vi "Resize.Align Child Tab Ctrl within Parent Tab Ctrl.vi"(4 "Child Ref Pos":T1(ring), 5 "dY":i32, 6 "Parent Ref Pos":T1(ring), 7 "dX":i32, 8 "error in":errorcluster, 10 "Child Tab Ctrl":refnum<vi>, 11 "Parent Tab Ctrl":refnum<vi>) -> (0 "error out":errorcluster, 2 "Child Tab Ctrl Out":refnum<vi>, 3 "Parent Tab Ctrl Out":refnum<vi>)   [LabVIEW 2024, in "EQMF.lvlib" / "Controls.lvlib"]
doc: "This VI aligns a tab control (child) within another tab control (parent).\nThe inner control is moved to within Dx and Dy distance (in pixels) from the referenced corners specified by the inputs Parent Ref Pos and Child Ref Pos.\n\nINPUTS:\n<B>dX</B> - The delta X position.\n<B>dY</B> - The delta Y position.\n<B>Parent Tab Ctrl</B> - Control of the parent tab.\n<B>Child Tab Ctrl</B> - Control of the child tab.\n<B>Parent Ref Pos</B> - An enumerator specifying the corner that is to be aligned.\n<B>Child Ref Pos</B> - An enumerator specifying the corner that is to be aligned.\n\nOUTPUTS:\n<B>Parent Tab Ctrl</B> - Duplicate control of the parent tab.\n<B>Child Tab Ctrl</B> - Duplicate control of the child tab.\n\nERRORS: \nAn error will be generated if one of the controls are the incorrect type or if the control reference is invalid."
uses:
  Controls.lvlib
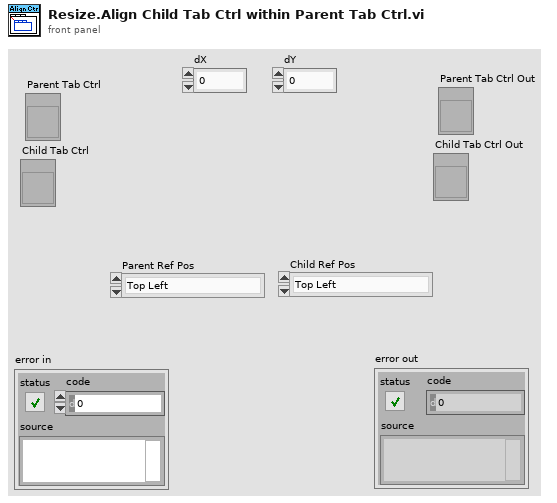
[diagram p1: front panel]
types:
  T1 = enum16{"Top Left", "Top Right", "Bottom Left", "Bottom Right"}
  T2 = typedef "EQMF.lvlib/Controls.lvlib/Ctrl.Object Position Info.ctl" = cluster{"Left":i32, "Right":i32, "Width":i32, "Top":i32, "Bottom":i32, "Height":i32}
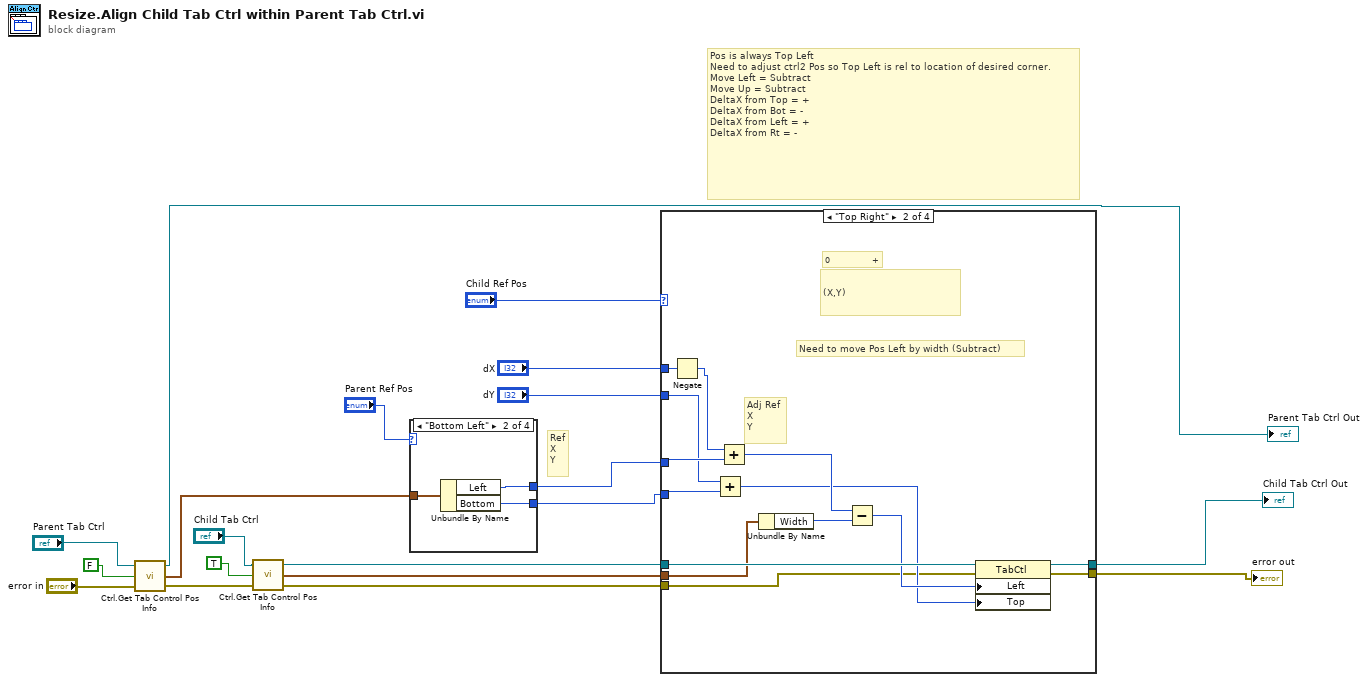
[diagram p0: block diagram]
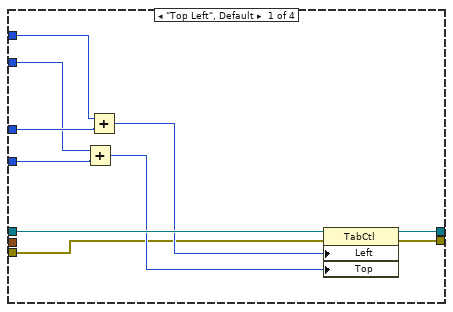
[diagram p2: hidden frame]
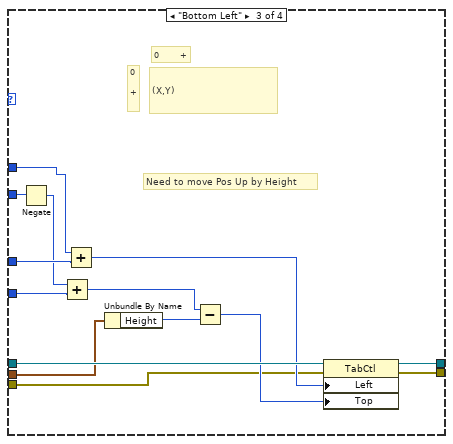
[diagram p3: hidden frame]
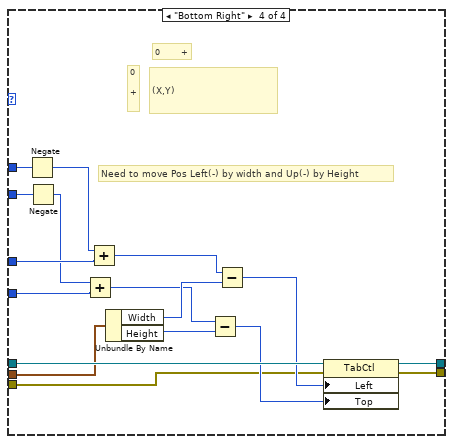
[diagram p4: hidden frame]
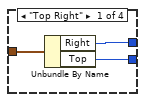
[diagram p5: hidden frame]
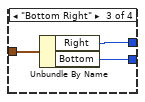
[diagram p6: hidden frame]
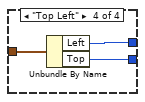
[diagram p7: hidden frame]
diagram:
  # "Pos is always Top Left\nNeed to adjust ctrl2 Pos so Top Left is rel to location of desired corner.\nMove Left = Subtract\nMove Up = Subtract\nDeltaX from Top = +\nDeltaX from Bot = -\nDeltaX from Left = +\nDeltaX from Rt = -"
  # "Ref\nX\nY"
  n1 = call "Ctrl.Get Tab Control Pos Info.vi"("error in"="error in", "Include Tab Height"=FALSE, "TabCtl Ref"="Parent Tab Ctrl") -> ("error out"=w4:errorcluster, "Pos Info"=w16:T2, "TabCtl Ref Out"=→"Parent Tab Ctrl Out":refnum<vi>)
  n2 = call "Ctrl.Get Tab Control Pos Info.vi"("error in"=w4, "Include Tab Height"=TRUE, "TabCtl Ref"="Child Tab Ctrl") -> ("error out"=w3:errorcluster, "Pos Info"=w14:T2, "TabCtl Ref Out"=w13:refnum<vi>)
  n3 = case shown="\"Bottom Left\"" "Parent Ref Pos" {
    tunnel: w16 -> [w22 w25 w28 w31]
    tunnel: [w21 w24 w27 w30] -> w11
    tunnel: [w20 w23 w26 w29] -> w12
    frame "Top Right" {
      n4 = Unbundle By Name(w22) -> ("Right"=w21:i32, "Top"=w20:i32)
    }
    frame "Bottom Left" {
      n5 = Unbundle By Name(w25) -> ("Left"=w24:i32, "Bottom"=w23:i32)
    }
    frame "Bottom Right" {
      n6 = Unbundle By Name(w28) -> ("Right"=w27:i32, "Bottom"=w26:i32)
    }
    frame "Top Left" {
      n7 = Unbundle By Name(w31) -> ("Left"=w30:i32, "Top"=w29:i32)
    }
  }
  n8 = case shown="\"Top Right\"" "Child Ref Pos" {
    tunnel: w14 -> [_ w52 w66 w83]
    tunnel: w11 -> [w38 w48 w60 w77]
    tunnel: w12 -> [w37 w49 w62 w78]
    tunnel: w13 -> [w41 w55 w69 w86]
    tunnel: [w40 w54 w68 w85] -> w2
    tunnel: [w39 w53 w67 w84] -> w6
    tunnel: "dY" -> [w35 w47 w58 w72]
    tunnel: "dX" -> [w36 w44 w63 w74]
    tunnel: w3 -> [w32 w42 w56 w70]
    frame "Top Left", Default {
      n9 = Add(x=w35, y=w37) -> (x+y=w33:i32)
      n10 = Add(x=w36, y=w38) -> (x+y=w34:i32)
      n11 = property class="TabCtl"(reference=w41, error in=w32, "Left"=w34, "Top"=w33) -> (reference out=w40:refnum<vi>, error out=w39:errorcluster)
    }
    frame "Top Right" {
      # "Adj Ref\nX\nY"
      # "0              +"
      # "Need to move Pos Left by width (Subtract)"
      # "(X,Y)"
      n12 = Negate(x=w44) -> (-x=w43:i32)
      n13 = Add(x=w47, y=w49) -> (x+y=w45:i32)
      n14 = Add(x=w43, y=w48) -> (x+y=w46:i32)
      n15 = Unbundle By Name(w52) -> ("Width"=w51:i32)
      n16 = Subtract(x=w46, y=w51) -> (x-y=w50:i32)
      n17 = property class="TabCtl"(reference=w55, error in=w42, "Left"=w50, "Top"=w45) -> (reference out=w54:refnum<vi>, error out=w53:errorcluster)
    }
    frame "Bottom Left" {
      # "0       +"
      # "0\n\n+"
      # "Need to move Pos Up by Height"
      # "(X,Y)"
      n18 = Negate(x=w58) -> (-x=w57:i32)
      n19 = Add(x=w57, y=w62) -> (x+y=w61:i32)
      n20 = Add(x=w63, y=w60) -> (x+y=w59:i32)
      n21 = Unbundle By Name(w66) -> ("Height"=w65:i32)
      n22 = Subtract(x=w61, y=w65) -> (x-y=w64:i32)
      n23 = property class="TabCtl"(reference=w69, error in=w56, "Left"=w59, "Top"=w64) -> (reference out=w68:refnum<vi>, error out=w67:errorcluster)
    }
    frame "Bottom Right" {
      # "0       +"
      # "0\n\n+"
      # "Need to move Pos Left(-) by width and Up(-) by Height"
      # "(X,Y)"
      n24 = Negate(x=w74) -> (-x=w73:i32)
      n25 = Negate(x=w72) -> (-x=w71:i32)
      n26 = Add(x=w71, y=w78) -> (x+y=w76:i32)
      n27 = Add(x=w73, y=w77) -> (x+y=w75:i32)
      n28 = Unbundle By Name(w83) -> ("Width"=w80:i32, "Height"=w82:i32)
      n29 = Subtract(x=w76, y=w82) -> (x-y=w81:i32)
      n30 = Subtract(x=w75, y=w80) -> (x-y=w79:i32)
      n31 = property class="TabCtl"(reference=w86, error in=w70, "Left"=w79, "Top"=w81) -> (reference out=w85:refnum<vi>, error out=w84:errorcluster)
    }
  }
  "error out" <- w6
  "Child Tab Ctrl Out" <- w2
